vi "test-linear-filter-output-test-02D.vi"() -> (3 "Passed":bool)   [LabVIEW 2019]
uses:
  <vilib>/ptbypt/NI_PtbyPt.lvlib
  <vilib>/Rock Robotics/WPI/ThirdParty/JAS_Junk/TrajLib/Trajectory_Library.lvlib
panel:
  out "Output 2":dbl
  out "Array":dbl[](array[numeric])
  out "Output":dbl
  out "Waveform Chart":cluster{"Output":dbl, "Output":dbl, dbl}(graph)
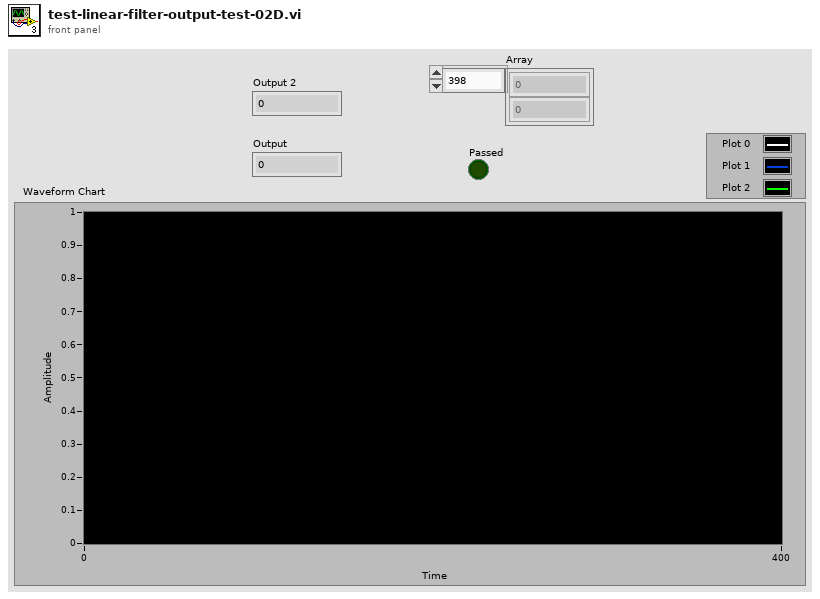
[diagram p1: front panel]
types:
  T1 = typedef "Trajectory_Library.lvlib/LINEAR_FILTER.ctl" = cluster{"InputGains":dbl[], "OutputGains":dbl[], "Inputs":dbl[], "Outputs":dbl[], "InGainCount":i32, "OutGainCount":i32}
  T2 = cluster{"Output":dbl, "Output":dbl, "Output":dbl}
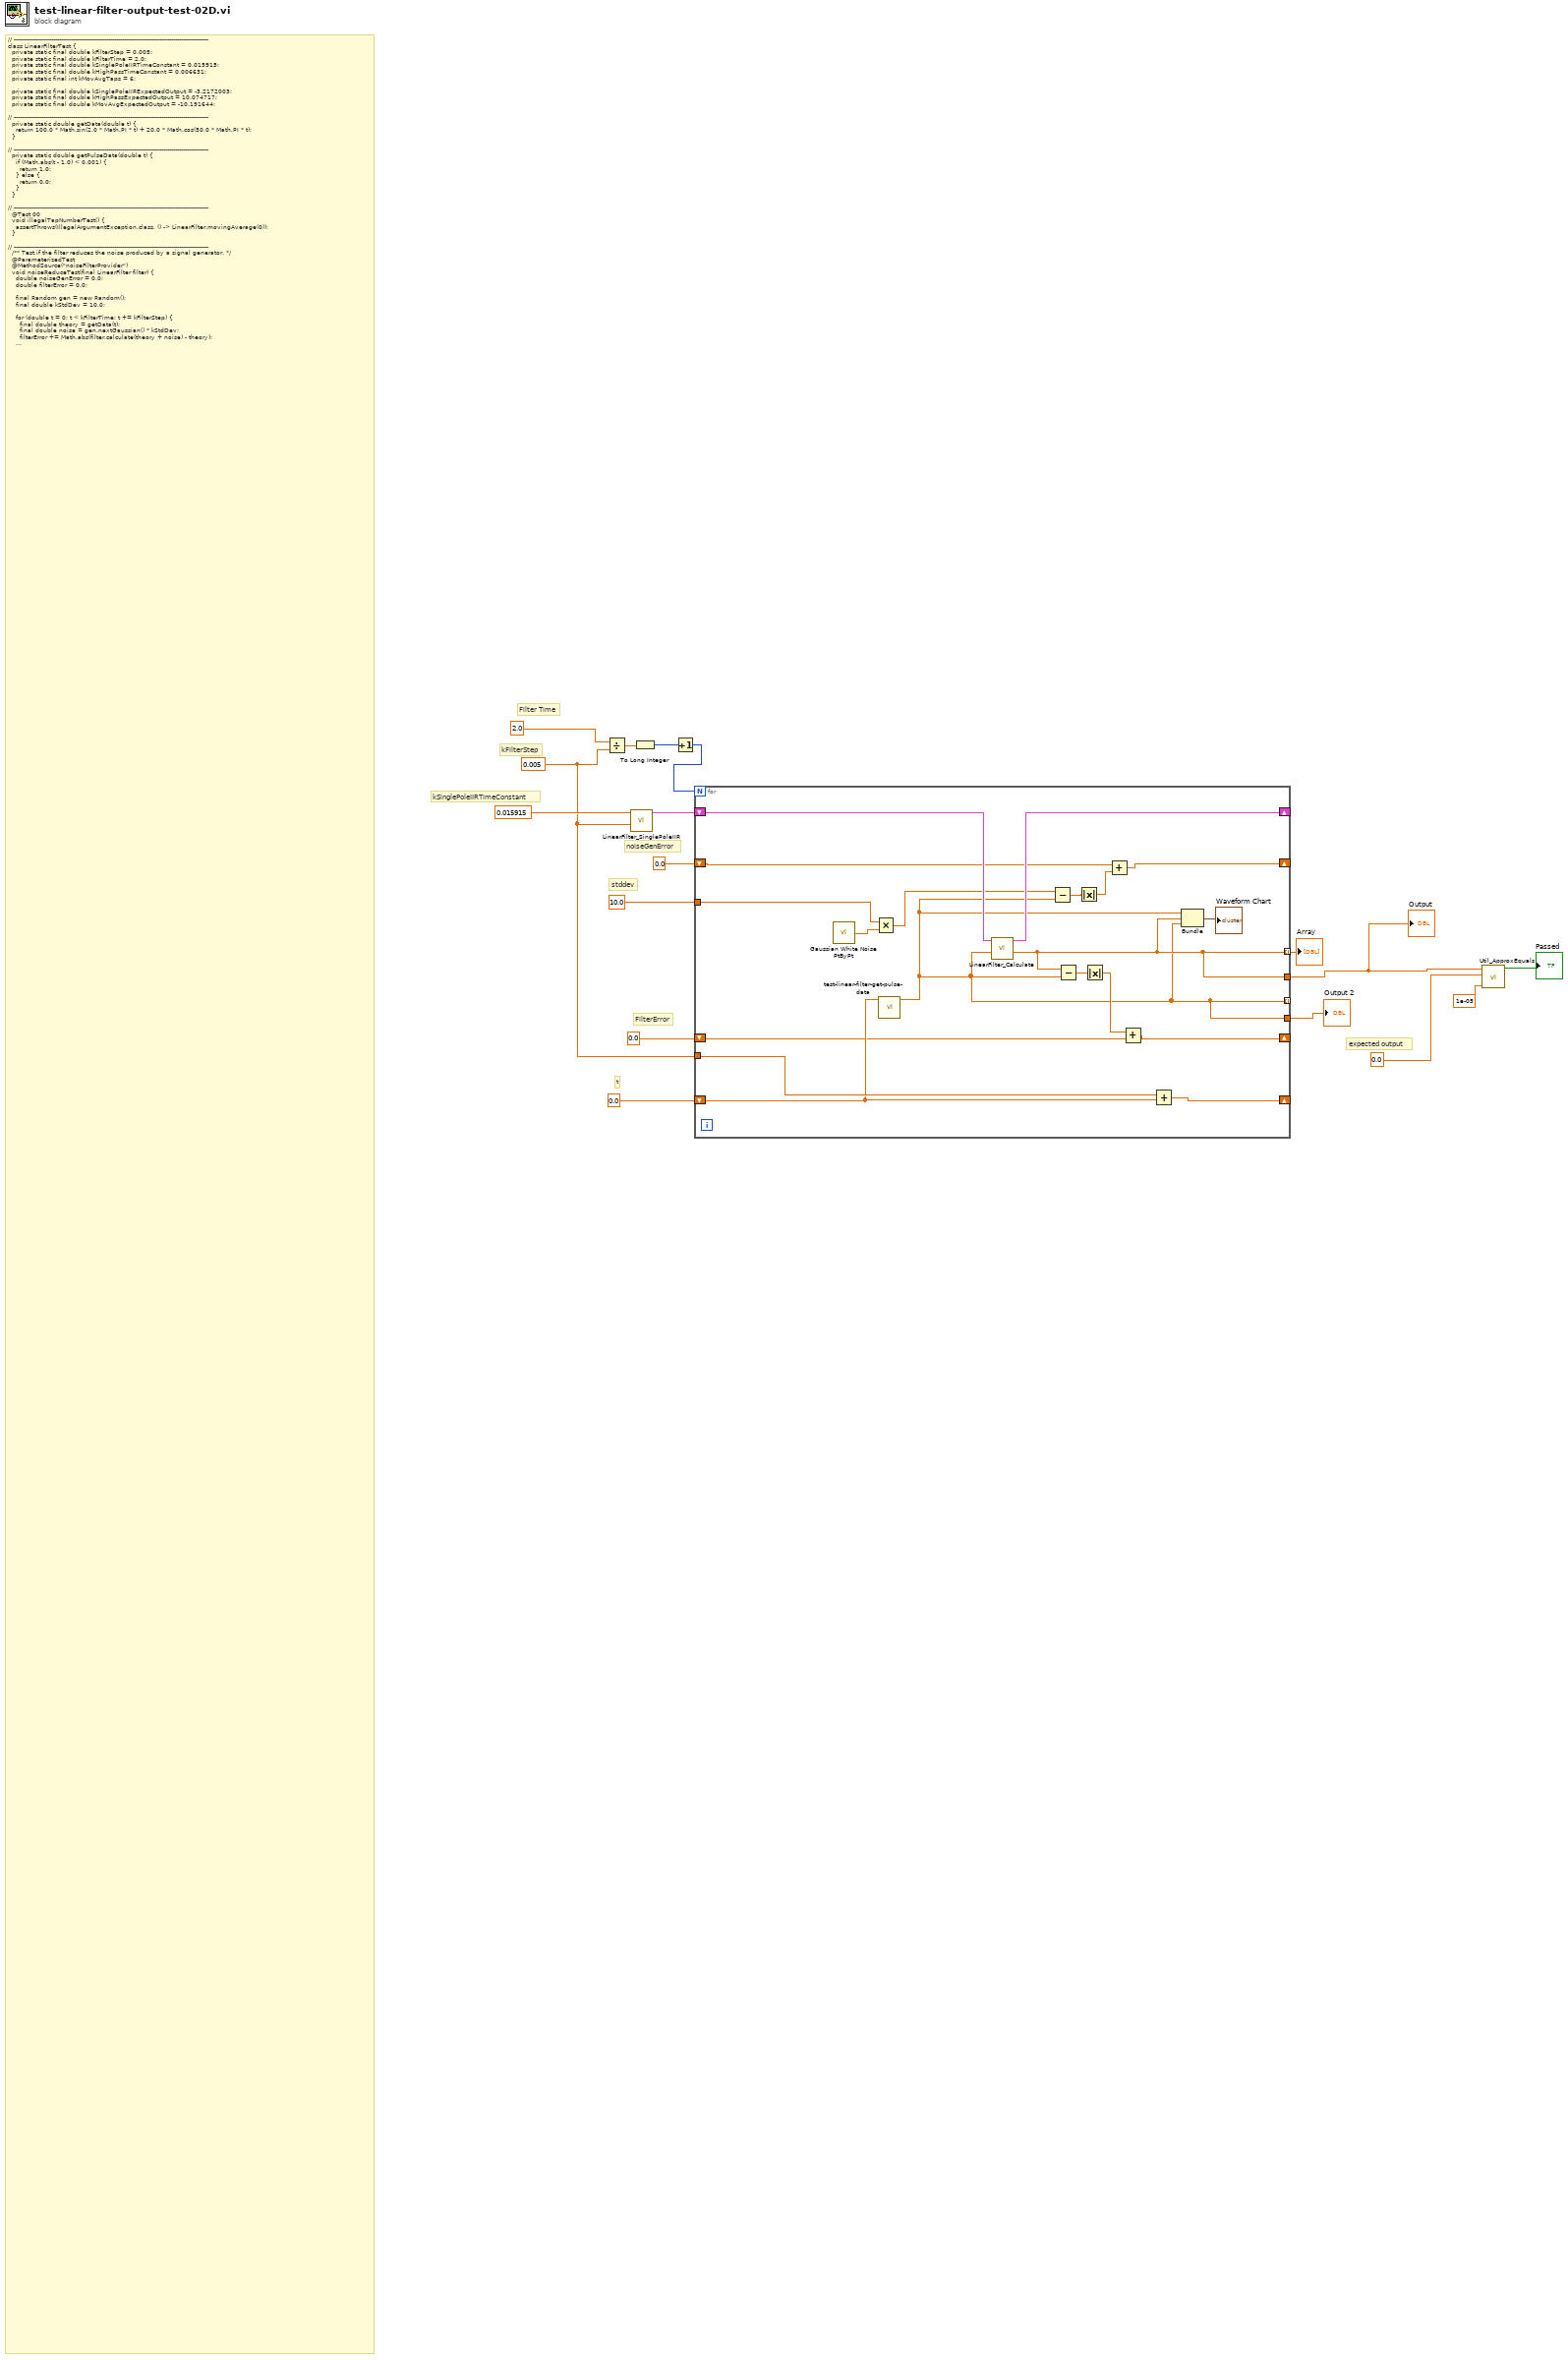
[diagram p0: block diagram]
diagram:
  w12 = 0.005
  # "expected output"
  # "kSinglePoleIIRTimeConstant"
  # "stddev"
  # "t"
  # "kFilterStep"
  # "Filter Time"
  # "FilterError"
  # "noiseGenError"
  # "// ---------------------------------------------------------------------------------------------------\nclass LinearFilterTest {\n  private static final double kFilterStep = 0.005;\n  private static final double kFilterTime = 2.0;\n  private static final double kSinglePoleIIRTimeConstant = 0.015915;\n  private static final double kHighPassTimeConstant = 0.006631;\n  private static final int kMovAvgTaps = 6;\n\n  private static final double kSinglePoleIIRExpectedOutput = -3.2172003;\n  private static final double kHighPassExpectedOutput = 10.074717;\n  private static final double kMovAvgExpectedOutput = -10.191644;\n\n// ---------------------------------------------------------------------------------------------------\n  private static double getData(double t) {\n    return 100.0 * Math.sin(2.0 * Math.PI * t) + 20.0 * Math.cos(50.0 * Math.PI * t);\n  }\n\n// ---------------------------------------------------------------------------------------------------\n  private static double getPulseData(double t) {\n    if (Math.abs(t - 1.0) < 0.001) {\n      return 1.0;\n    } else {\n      return 0.0;\n    }\n  }\n\n// ---------------------------------------------------------------------------------------------------\n  @Test 00\n  void illegalTapNumberTest() {\n    assertThrows(IllegalArgumentException.class, () -> LinearFilter.movingAverage(0));\n  }\n\n// ---------------------------------------------------------------------------------------------------\n  /** Test if the filter reduces the noise produced by a signal generator. */\n  @ParameterizedTest\n  @MethodSource(\"noiseFilterProvider\")\n  void noiseReduceTest(final LinearFilter filter) {\n    double noiseGenError = 0.0;\n    double filterError = 0.0;\n\n    final Random gen = new Random();\n    final double kStdDev = 10.0;\n\n    for (double t = 0; t < kFilterTime; t += kFilterStep) {\n      final double theory = getData(t);\n      final double noise = gen.nextGaussian() * kStdDev;\n      filterError += Math.abs(filter.calculate(theory + noise) - theory);\n      noiseGenError += Math.abs(noise - theory);\n    }\n\n    assertTrue(\n        noiseGenError > filterError,\n        \"Filter should have reduced noise accumulation from \"\n            + noiseGenError\n            + \" but failed. The filter error was \"\n            + filterError);\n  }\n\n  static Stream<LinearFilter> noiseFilterProvider() {\n    return Stream.of(\n        LinearFilter.singlePoleIIR(kSinglePoleIIRTimeConstant, kFilterStep),\n        LinearFilter.movingAverage(kMovAvgTaps));\n  }\n\n// ---------------------------------------------------------------------------------------------------\n  /** Test if the linear filters produce consistent output for a given data set. */\n  @ParameterizedTest\n  @MethodSource(\"outputFilterProvider\")\n  void outputTest(\n                    final LinearFilter filter, \n                   final DoubleFunction<Double> data, \n                    final double expectedOutput) {\n\n\n    double filterOutput = 0.0;\n    for (double t = 0.0; t < kFilterTime; t += kFilterStep) {\n      filterOutput = filter.calculate(data.apply(t));\n    }\n\n    assertEquals(expectedOutput, filterOutput, 5e-5, \"Filter output was incorrect.\");\n  }\n\n  static Stream<Arguments> outputFilterProvider() {\n    return Stream.of(\n        arguments(\n            LinearFilter.singlePoleIIR(kSinglePoleIIRTimeConstant, kFilterStep),\n            (DoubleFunction<Double>) LinearFilterTest::getData,\n            kSinglePoleIIRExpectedOutput),\n        arguments(\n            LinearFilter.highPass(kHighPassTimeConstant, kFilterStep),\n            (DoubleFunction<Double>) LinearFilterTest::getData,\n            kHighPassExpectedOutput),\n        arguments(\n            LinearFilter.movingAverage(kMovAvgTaps),\n            (DoubleFunction<Double>) LinearFilterTest::getData,\n            kMovAvgExpectedOutput),\n        arguments(\n            LinearFilter.movingAverage(kMovAvgTaps),\n            (DoubleFunction<Double>) LinearFilterTest::getPulseData,\n            0.0));\n  }\n\n// ---------------------------------------------------------------------------------------------------\n  /** Test backward finite difference. */\n  @Test\n  void backwardFiniteDifferenceTest() {\n    double h = 0.005;\n\n    assertResults(\n        1,\n        2,\n        // f(x) = x²\n        (double x) -> x * x,\n        // df/dx = 2x\n        (double x) -> 2.0 * x,\n        h,\n        -20.0,\n        20.0);\n\n    assertResults(\n        1,\n        2,\n        // f(x) = sin(x)\n        (double x) -> Math.sin(x),\n        // df/dx = cos(x)\n        (double x) -> Math.cos(x),\n        h,\n        -20.0,\n        20.0);\n\n    assertResults(\n        1,\n        2,\n        // f(x) = ln(x)\n        (double x) -> Math.log(x),\n        // df/dx = 1 / x\n        (double x) -> 1.0 / x,\n        h,\n        1.0,\n        20.0);\n\n    assertResults(\n        2,\n        4,\n        // f(x) = x²\n        (double x) -> x * x,\n        // d²f/dx² = 2\n        (double x) -> 2.0,\n        h,\n        -20.0,\n        20.0);\n\n    assertResults(\n        2,\n        4,\n        // f(x) = sin(x)\n        (double x) -> Math.sin(x),\n        // d²f/dx² = -sin(x)\n        (double x) -> -Math.sin(x),\n        h,\n        -20.0,\n        20.0);\n\n    assertResults(\n        2,\n        4,\n        // f(x) = ln(x)\n        (double x) -> Math.log(x),\n        // d²f/dx² = -1 / x²\n        (double x) -> -1.0 / (x * x),\n        h,\n        1.0,\n        20.0);\n  }\n\n// ---------------------------------------------------------------------------------------------------\n  /**\n   * Helper for checking results of backward finite difference.\n   *\n   * @param derivative The order of the derivative.\n   * @param samples The number of sample points.\n   * @param f Function of which to take derivative.\n   * @param dfdx Derivative of f.\n   * @param h Sample period in seconds.\n   * @param min Minimum of f's domain to test.\n   * @param max Maximum of f's domain to test.\n   */\n  void assertResults(\n      int derivative,\n      int samples,\n      DoubleFunction<Double> f,\n      DoubleFunction<Double> dfdx,\n      double h,\n      double min,\n      double max) {\n    var filter = LinearFilter.backwardFiniteDifference(derivative, samples, h);\n\n    for (int i = (int) (min / h); i < (int) (max / h); ++i) {\n      // Let filter initialize\n      if (i < (int) (min / h) + samples) {\n        filter.calculate(f.apply(i * h));\n        continue;\n      }\n\n      // The order of accuracy is O(h^(N - d)) where N is number of stencil\n      // points and d is order of derivative\n      assertEquals(\n          dfdx.apply(i * h),\n          filter.calculate(f.apply(i * h)),\n          10.0 * Math.pow(h, samples - derivative));\n    }\n  }\n}"
  n1 = Divide(x=2.0, y=w12) -> (x/y=w17:dbl)
  n2 = call <vilib>:"LinearFilter_SinglePoleIIR.vi"("SamplePeriod"=w12, "TimeConstant"=0.015915) -> ("LINEAR_FILTER"=w11:T1)  [unwired: 8 in, 1 out]
  n3 = To Long Integer(number=w17) -> (32bit integer=w2:i32)
  n4 = Increment(x=w2) -> (x+1=w1:i32)
  n5 = for {
    N: w1 -> [_]
    shift-right: [w35] -> _
    shift-left: 0.0 -> [w34]
    tunnel: w12 -> [w36]
    tunnel: 10.0 -> [w32]
    shift-right: [w30] -> _
    shift-left: w11 -> [w31]
    tunnel: [w18] -> _ mode=indexing
    tunnel: [w19] -> w4 mode=indexing
    shift-right: [w27] -> _
    shift-left: 0.0 -> [w26]
    shift-right: [w23] -> _
    shift-left: 0.0 -> [w22]
    tunnel: [w19] -> w8
    tunnel: [w18] -> w3
    n6 = call <vilib>:"Gaussian White Noise PtByPt.vi"() -> ("Gaussian white noise"=w33:dbl)  [unwired: 3 in]
    n7 = Multiply(x=w32, y=w33) -> (x*y=w25:dbl)
    n8 = call "test-linear-filter-get-pulse-data.vi"("T"=w34) -> ("Output"=w18:dbl)  [unwired: 10 in]
    n9 = call <vilib>:"LinearFilter_Calculate.vi"("Input"=w18, "In LINEAR_FILTER"=w31) -> ("Output"=w19:dbl, "Out LINEAR_FILTER"=w30:T1)  [unwired: 8 in]
    n10 = Subtract(x=w25, y=w18) -> (x-y=w24:dbl)
    n11 = Subtract(x=w19, y=w18) -> (x-y=w29:dbl)
    n12 = Absolute Value(x=w24) -> (abs(x)=w21:dbl)
    n13 = Absolute Value(x=w29) -> (abs(x)=w28:dbl)
    n14 = Add(x=w22, y=w21) -> (x+y=w23:dbl)
    n15 = Add(x=w28, y=w26) -> (x+y=w27:dbl)
    n16 = Add(x=w36, y=w34) -> (x+y=w35:dbl)
    n17 = Bundle("Output"=w18, "Output"=w19, "Output"=w18) -> (→"Waveform Chart":T2)  [unwired: 1 in]
  }
  "Output" <- w8
  "Array" <- w4
  "Output 2" <- w3
  n18 = call <vilib>:"Util_ApproxEquals.vi"("Tolerance"=1e-05, "Value 2"=0.0, "Value 1"=w8) -> ("ApproxEquals"=→"Passed":bool)  [unwired: 8 in]
